vi "BuildMeasArray.vi"(1 "#Steps":i32, 2 "Stop":dbl, 3 "Start":dbl) -> (0 "MeasArray":dbl[](array[numeric]))   [LabVIEW 2017]
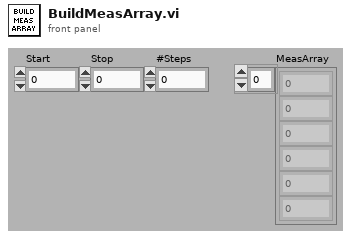
[diagram p1: front panel]
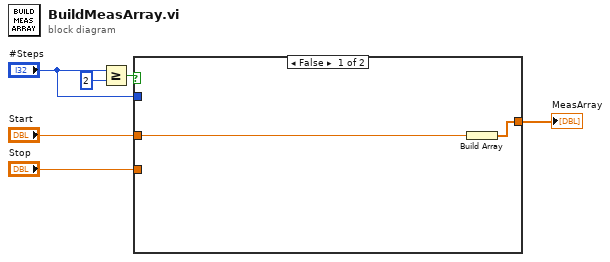
[diagram p0: block diagram]
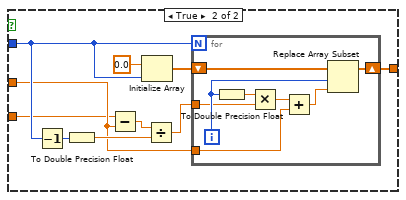
[diagram p2: hidden frame]
diagram:
  n1 = Greater Or Equal?(x="#Steps", y=2 ("x")) -> (x >= y?=w5:bool)
  n2 = case shown="False" w5 {
    tunnel: [w8 w18] -> w6
    tunnel: "#Steps" -> [_ w11]
    tunnel: "Start" -> [w7 w10]
    tunnel: "Stop" -> [_ w9]
    frame False {
      n3 = Build Array(w7) -> (w8:dbl[])
    }
    frame True {
      n4 = Decrement(x=w11) -> (x-1=w12:i32)
      n5 = To Double Precision Float(number=w12) -> (double precision float=w14:dbl)
      n6 = Subtract(x=w9, y=w10) -> (x-y=w15:dbl)
      n7 = Initialize Array(0.0 ("element"), w11) -> (w16:dbl[])
      n8 = Divide(x=w15, y=w14) -> (x/y=w13:dbl)
      n9 = for {
        N: w11 -> [_]
        shift-right: [w25] -> w18
        shift-left: w16 -> [w26]
        tunnel: w13 -> [w22]
        tunnel: w10 -> [w19]
        i -> [w24]
        n10 = To Double Precision Float(number=w24) -> (double precision float=w23:dbl)
        n11 = Multiply(x=w23, y=w22) -> (x*y=w21:dbl)
        n12 = Add(x=w21, y=w19) -> (x+y=w20:dbl)
        n13 = Replace Array Subset(array=w26, new element=w20, index=w24) -> (w25:dbl[])
      }
    }
  }
  "MeasArray" <- w6
